vi "database_connection_write_G1.vi"(5 "ODBC data source name":string="amrc_monitoring", 6 "error in (no error)":errorcluster, 7 "G1?":u32, 8 "current time":timestamp, 9 "data 2":dbl[](array[numeric]), 10 "Machine Data":T1, 11 "Machine type":string) -> (3 "error out":errorcluster)   [LabVIEW 2014]
uses:
  <vilib>/addons/database/Connection.llb/DB Tools Open Connec (String).vi
  <vilib>/addons/database/Connection.llb/Conn Execute.vi
  <vilib>/addons/database/Recordset.llb/Rec Destroy - Connection.vi
  <vilib>/addons/database/NI_Database_API.lvlib
panel:
  out "concatenated string":string
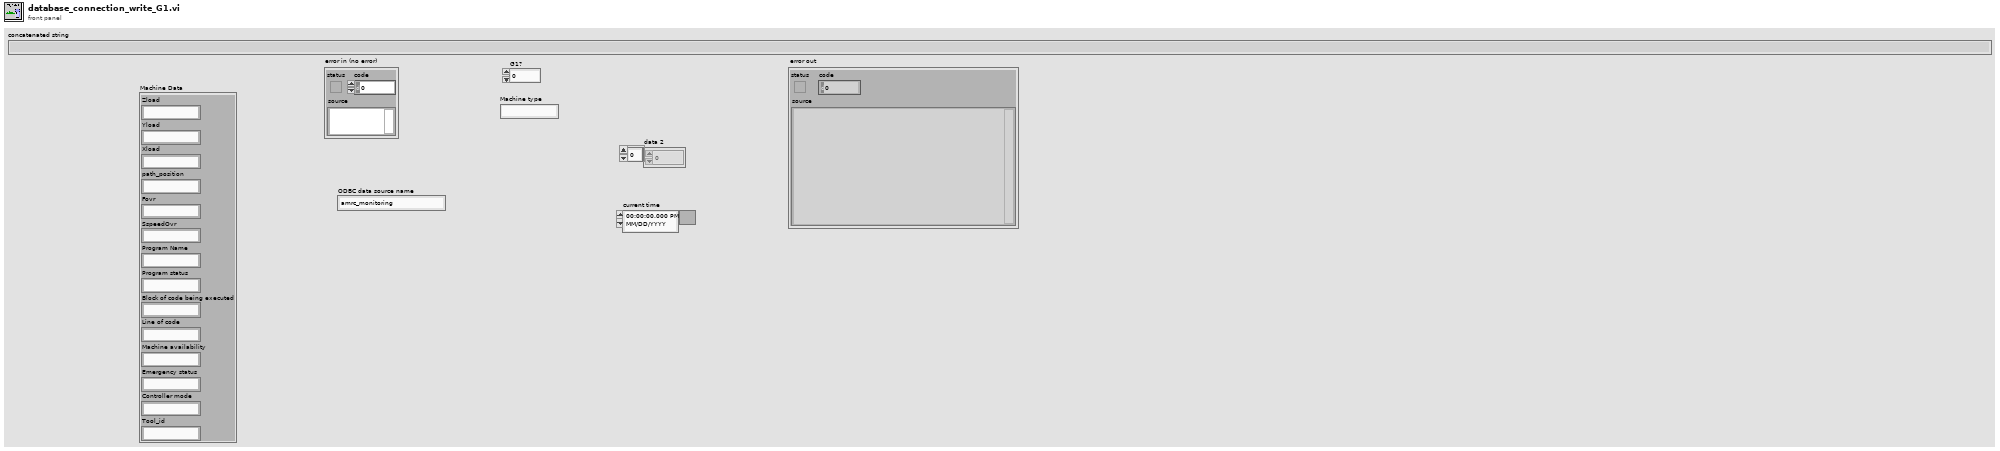
[diagram p1: front panel]
types:
  T1 = cluster{"Zload":string, "Yload":string, "Xload":string, "path_position":string, "Fovr":string, "SspeedOvr":string, "Program Name":string, "Program status":string, "Block of code being executed":string, "Line of code":string, "Machine availability":string, "Emergency status":string, "Controller mode":string, "Tool_id":string}
  T2 = typedef "NI_Database_API.lvlib/Conn ObjectReference.ctl" = refnum<k1>
  T3 = typedef "NI_Database_API.lvlib/Rec ObjectReference.ctl" = refnum<k1>
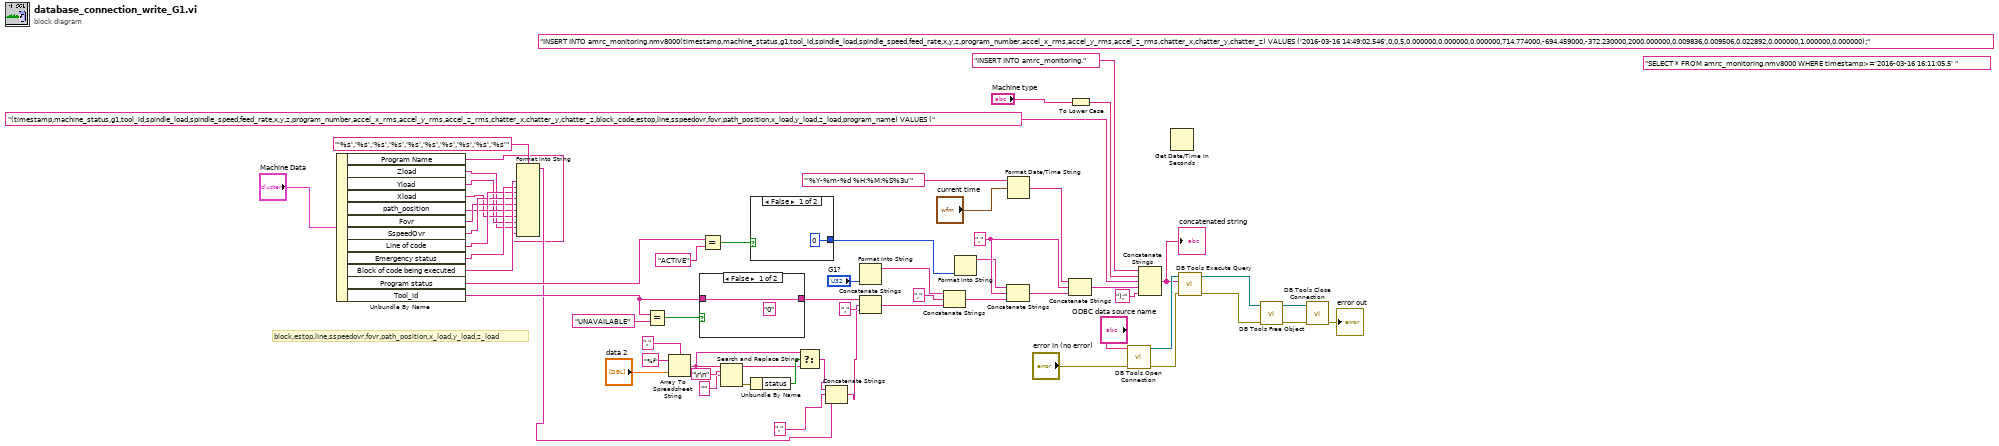
[diagram p0: block diagram]
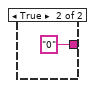
[diagram p2: hidden frame]
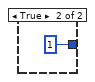
[diagram p3: hidden frame]
diagram:
  w35 = "," ("string")
  (unwired) "SELECT * FROM amrc_monitoring.nmv8000 WHERE timestamp>='2016-03-16 16:11:05.5' " ("SQL query")
  (unwired) "INSERT INTO amrc_monitoring.nmv8000(timestamp,machine_status,g1,tool_id,spindle_load,spindle_speed,feed_rate,x,y,z,program_number,accel_x_rms,accel_y_rms,accel_z_rms,chatter_x,chatter_y,chatter_z) VALUES ('2016-03-16 14:49:02.546',0,0,5,0.000000,0.000000,0.000000,714.774000,-694.459000,-372.230000,2000.000000,0.009836,0.009506,0.022892,0.000000,1.000000,0.000000);" ("SQL query")
  # "block,estop,line,sspeedovr,fovr,path_position,x_load,y_load,z_load"
  n1 = Unbundle By Name("Machine Data") -> ("Program Name"=w1:string, "Zload"=w8:string, "Yload"=w9:string, "Xload"=w10:string, "path_position"=w11:string, "Fovr"=w12:string, "SspeedOvr"=w13:string, "Line of code"=w14:string, "Emergency status"=w15:string, "Block of code being executed"=w16:string, "Program status"=w52:string, "Tool_id"=w46:string)
  n2 = Format Into String(format string="'%s','%s','%s','%s','%s','%s','%s','%s','%s','%s'", w16, w15, w14, w13, w12, w11, w10, w9, w8, w1) -> (resulting string=w5:string)  [unwired: 2 in, 1 out]
  n3 = Equal?(x=w46, y="UNAVAILABLE") -> (x = y?=w47:bool)
  n4 = Array To Spreadsheet String(delimiter (Tab)=",", array="data 2", 3:"%f" ("format string")) -> (spreadsheet string=w26:string)
  n5 = case shown="False" w47 {
    tunnel: w46 -> [w62 _]
    tunnel: [w62 "0"] -> w45
    frame False {
      (unwired) "0"
    }
    frame True {
    }
  }
  n6 = Equal?(x=w52, y="ACTIVE") -> (x = y?=w50:bool)
  n7 = Search and Replace String(input string=w26, search string="\r\n", replace string="" ("replace string (\"\")")) -> (result string=w27:string, error out=w29:errorcluster)  [unwired: 5 in, 2 out]
  n8 = case shown="False" w50 {
    tunnel: [0 1] -> w49
    frame False {
    }
    frame True {
    }
  }
  n9 = Unbundle By Name(w29) -> ("status"=w28:bool)
  n10 = Select(t=w26, s=w28, f=w27) -> (s? t:f=w3:string)
  n11 = Concatenate Strings(w3, "," ("string"), w5) -> (w2:string)
  n12 = Format Into String("G1?") -> (resulting string=w42:string)  [unwired: 3 in, 1 out]
  n13 = Concatenate Strings(w45, "," ("string"), w2) -> (w41:string)
  n14 = Concatenate Strings(w42, "," ("string"), w41) -> (w37:string)
  n15 = Format Into String(w49) -> (resulting string=w33:string)  [unwired: 3 in, 1 out]
  n16 = Concatenate Strings(w33, w35, w37) -> (w36:string)
  n17 = Format Date/Time String(time format string (%c)="'%Y-%m-%d %H:%M:%S%3u'", seconds (now)="current time") -> (date/time string=w34:string)  [unwired: 1 in]
  n18 = Concatenate Strings(w34, w35, w36) -> (w32:string)
  n19 = To Lower Case(string="Machine type") -> (all lower case string=w23:string)
  n20 = call-poly <vilib>:"DB Tools Open Connection.vi"("error in (no error)"="error in (no error)", "connection information"="ODBC data source name") -> ("error out"=w60:errorcluster, "connection reference"=w61:T2)  [unwired: 6 in]
  n21 = Concatenate Strings("INSERT INTO amrc_monitoring." ("string"), w23, "(timestamp,machine_status,g1,tool_id,spindle_load,spindle_speed,feed_rate,x,y,z,program_number,accel_x_rms,accel_y_rms,accel_z_rms,chatter_x,chatter_y,chatter_z,block_code,estop,line,sspeedovr,fovr,path_position,x_load,y_load,z_load,program_name) VALUES (" ("string"), w32, ");" ("string")) -> (w4:string)
  "concatenated string" <- w4
  n22 = Get Date/Time In Seconds() -> ()  [unwired: 1 out]
  n23 = call-poly <vilib>:"DB Tools Execute Query.vi"("error in (no error)"=w60, "SQL query"=w4, "connection reference"=w61) -> ("error out"=w19:errorcluster, "recordset reference"=w18:T3)  [unwired: 5 in]
  n24 = call-poly <vilib>:"DB Tools Free Object.vi"("error in (no error)"=w19, "recordset reference"=w18) -> ("error out"=w59:errorcluster, "connection reference"=w58:T2)  [unwired: 8 in]
  n25 = call <vilib>:"DB Tools Close Connection.vi"("error in (no error)"=w59, "connection reference"=w58) -> ("error out"=→"error out":errorcluster)  [unwired: 5 in]
